vi "Cmd.ReadMessage.vi"(6 "Timeout [ms] (1000)":i32=1000, 8 "error in":errorcluster, 11 "cID in":refnum<k5>) -> (0 "error out":errorcluster, 2 "Message":string, 3 "cID out":refnum<k5>)   [LabVIEW 2016]
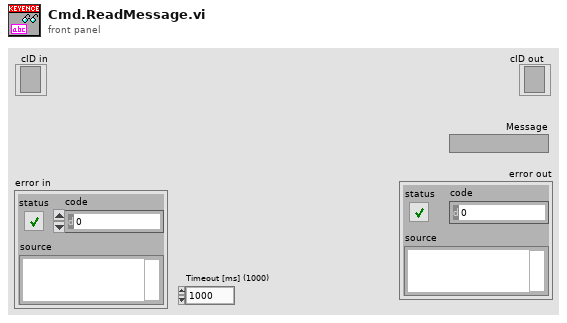
[diagram p1: front panel]
types:
  T1 = enum16{"Standard", "Buffered", "CRLF", "Immediate"}
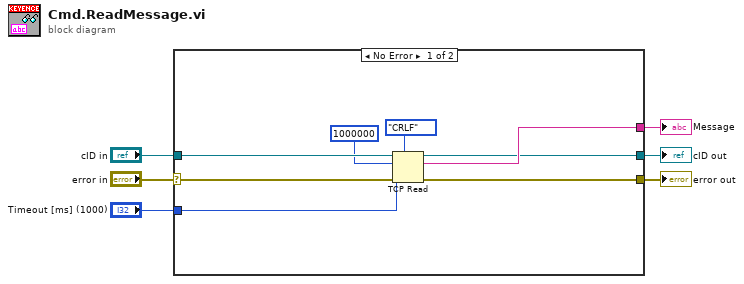
[diagram p0: block diagram]
diagram:
  n1 = case shown="No Error" "error in" {
    selector: "error in" -> [w11 w15]
    tunnel: "Timeout [ms] (1000)" -> [w8 _]
    tunnel: "cID in" -> [w14 w16]
    tunnel: [w7 w16] -> w3
    tunnel: [w10 w15] -> w2
    tunnel: [w9 _] -> w1
    frame No Error {
      n2 = TCP Read(connection ID=w14, bytes to read=1000000, error in (no error)=w11, 7:T1."CRLF" ("mode (standard)"), 9:w8) -> (connection ID out=w7:refnum<k5>, data out=w9:string, error out=w10:errorcluster)
    }
    frame Error {
    }
  }
  "cID out" <- w3
  "error out" <- w2
  "Message" <- w1
